vi "Vector-valued Function.vi"(1 "(x_1,...,x_n)":refnum<class "Dual.lvclass">[](array[class])) -> (0 "(f_1,...,f_n)":refnum<class "Dual.lvclass">[](array[class]))   [LabVIEW 2020, in "Examples.lvlib"]
doc: "f(x,y) =(x^2 + y^2 , 3xy)"
uses:
  classes/Dual/Dual.lvclass
  classes/Dual/Dual.lvclass/Dual.ctl
  6f97315e-7bac-45fb-98c9-d02ae5ecc296.vi
  72b3d7e6-e7b9-468f-a967-6ec54929e0e8.vi
  0232c1de-646f-48a7-bb7d-f7f53221b374.vi
  5b5ab934-7854-4bd5-a8aa-0cbb074ab388.vi
  1af88e31-763d-4e75-a921-d55d73349e85.vi
  6f97315e-7bac-45fb-98c9-d02ae5ecc296.vi/957074e8-cc3b-4647-8ff1-d975a744cd4e.vi
  classes/Dual/Write a and b.vi
  classes/Dual/Read a and b.vi
  72b3d7e6-e7b9-468f-a967-6ec54929e0e8.vi/b6499733-2759-4852-aa6b-3ec1516ef704.vi
  72b3d7e6-e7b9-468f-a967-6ec54929e0e8.vi/ce7907ec-4dc6-4618-8708-ad667a8e3a23.vi
  0232c1de-646f-48a7-bb7d-f7f53221b374.vi/b6499733-2759-4852-aa6b-3ec1516ef704.vi
  0232c1de-646f-48a7-bb7d-f7f53221b374.vi/ce7907ec-4dc6-4618-8708-ad667a8e3a23.vi
  5b5ab934-7854-4bd5-a8aa-0cbb074ab388.vi/957074e8-cc3b-4647-8ff1-d975a744cd4e.vi
  1af88e31-763d-4e75-a921-d55d73349e85.vi/6101d903-ff9f-41ff-96b8-b42400c258cc.vi
  1af88e31-763d-4e75-a921-d55d73349e85.vi/5aba97ba-e1f8-4e08-94e3-f0ae7cb31178.vi
  72b3d7e6-e7b9-468f-a967-6ec54929e0e8.vi/b6499733-2759-4852-aa6b-3ec1516ef704.vi/5957e011-cf56-4527-b6ed-13c3a4ca997b.vi
  classes/Dual/Write a.vi
  Examples.lvlib
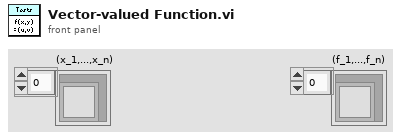
[diagram p1: front panel]
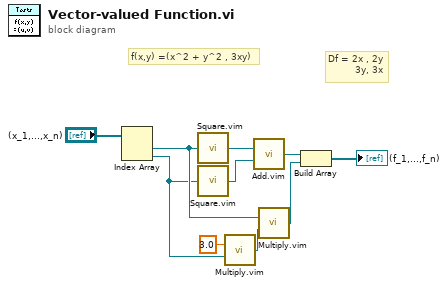
[diagram p0: block diagram]
diagram:
  # "Df = 2x , 2y\n         3y, 3x"
  # "f(x,y) =(x^2 + y^2 , 3xy)"
  n1 = Index Array(array="(x_1,...,x_n)") -> (element #1=w6:refnum<class "Dual.lvclass">, element #2=w1:refnum<class "Dual.lvclass">)  [unwired: 2 in]
  n2 = call "Square.vim"("x"=w6) -> ("x^2"=w10:refnum<class "Dual.lvclass">)
  n3 = call "Square.vim"("x"=w1) -> ("x^2"=w9:refnum<class "Dual.lvclass">)
  n4 = call "Multiply.vim"("x"=3.0 ("Double"), "y"=w1) -> ("x * y"=w5:refnum<class "Dual.lvclass">)  [unwired: 13 in]
  n5 = call "Add.vim"("x"=w10, "y"=w9) -> ("x + y"=w3:refnum<class "Dual.lvclass">)  [unwired: 13 in]
  n6 = call "Multiply.vim"("x"=w6, "y"=w5) -> ("x * y"=w4:refnum<class "Dual.lvclass">)  [unwired: 13 in]
  n7 = Build Array(w3, w4) -> (→"(f_1,...,f_n)":refnum<class "Dual.lvclass">[])
